vi "Set Motors.vi"(5 "Speed Multipliers":dbl=1.0, 6 "Face Joystick Axes":cluster{"X":dbl, "Y":dbl}, 7 "error in (no error)":errorcluster, 8 "Strafe Joystick Axes":cluster{"X":dbl, "Y":dbl}, 9 "Trigger Axes":cluster{"Left":dbl, "Right":dbl}, 10 "Speed Motors":T2[](array[typedef]), 11 "Position Motors":T2[](array[typedef])) -> (4 "error out":errorcluster)   [LabVIEW 2015]
uses:
  <vilib>/Rock Robotics/WPI/MotorControl/WPI_MotorControlDeviceRef.ctl
  <vilib>/Rock Robotics/WPI/MotorControl/WPI_MotorControlType.ctl
  <vilib>/Rock Robotics/SystemInterfaces/DIO/FPGA_DIOPWMChannel.ctl
  <vilib>/Rock Robotics/WPI/PWM/WPI_PWMDeadband.ctl
  <vilib>/Rock Robotics/WPI/CAN/Jaguar/SubVIs/WPI_CANJaguar_ControlMode.ctl
  <vilib>/Rock Robotics/WPI/CAN/TalonSRX/WPI_CANTalonSRX_APIControlMode.ctl
  Swerve Drive Published Globals.vi
  <vilib>/addons/control/pid/pid.llb/PID Control Input Filter (DBL).vi
  <vilib>/addons/control/pid/pid.llb/PID (DBL).vi
  <vilib>/addons/control/pid/NI_PID_pid.lvlib
panel:
  in  "Max Wheel Speed":dbl=20000.0
  in  "Angle (radians; 0 = right)":dbl
  in  "Face PID Gains":T1 {"derivative time (Td, min)" format="%.3f"; "integral time (Ti, min)" format="%.3f"; "proportional gain (Kc)" format="%.3f"}
  out "Speed Chart":cluster{dbl, "Encoder Velocity":dbl}[](graph)
  out "Position Chart":cluster{dbl, "Encoder Velocity":dbl}[](graph)
  out "Speed Cluster":T9 {"RR Speed" scale=-1.0..1.0; "RL Speed" scale=-1.0..1.0; "FR Speed" scale=-1.0..1.0; "FL Speed" scale=-1.0..1.0}
  out "Angle Cluster":T10 {"FL Angle" scale=3.1416..-3.1416; "FR Angle" scale=3.1416..-3.1416; "RR Angle" scale=3.1416..-3.1416; "RL Angle" scale=3.1416..-3.1416}
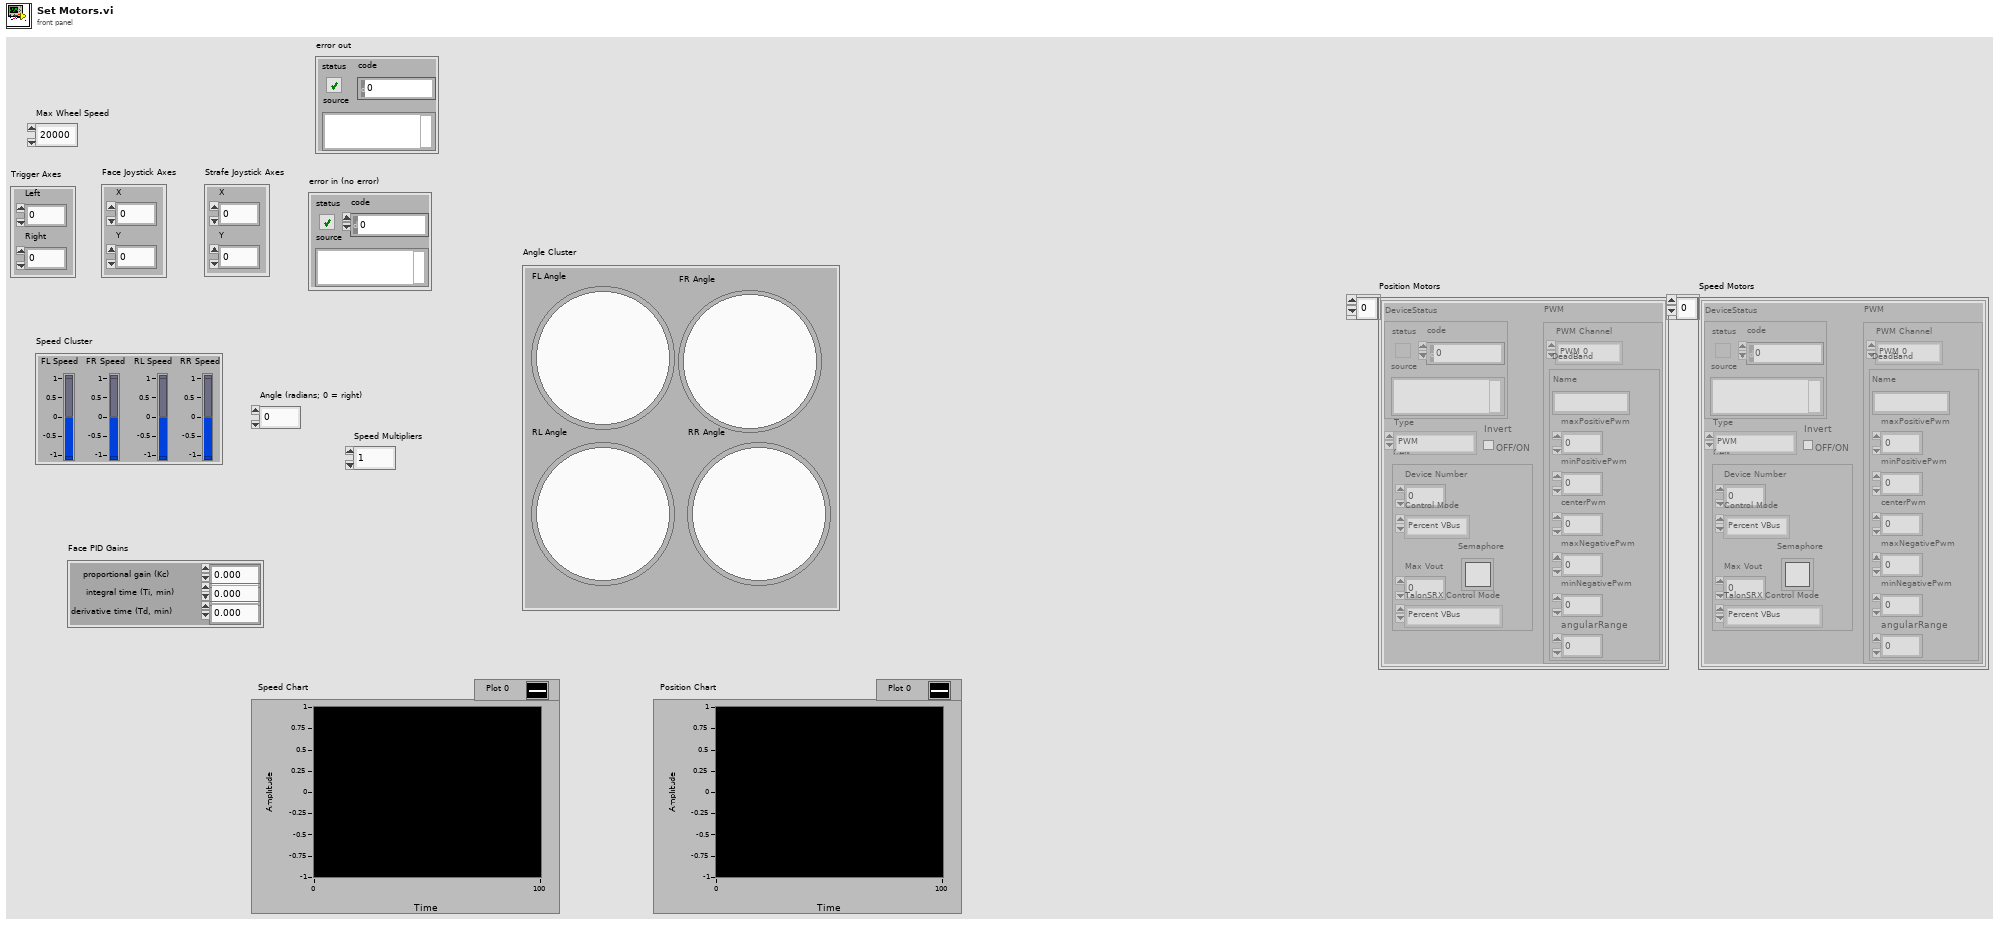
[diagram p1: front panel]
types:
  T1 = cluster{"proportional gain (Kc)":dbl, "integral time (Ti, min)":dbl, "derivative time (Td, min)":dbl}
  T2 = typedef "WPI_MotorControlDeviceRef.ctl" = cluster{"DeviceStatus":errorcluster, "Type":T3, "PWM":cluster{"PWM Channel":T4, "DeadBand":T5}, "CAN":cluster{"Device Number":u8, "Control Mode":T6, "Semaphore":T7, "Max Vout":dbl, "TalonSRX Control Mode":T8}, "Invert":bool}
  T3 = typedef "WPI_MotorControlType.ctl" = enum16{"PWM", "CAN", "CANTalonSRX"}
  T4 = typedef "FPGA_DIOPWMChannel.ctl" = enum8{"PWM 0", "PWM 1", "PWM 2", "PWM 3", "PWM 4", "PWM 5", "PWM 6", "PWM 7", "PWM 8", "PWM 9", "PWM MXP 0", "PWM MXP 1", "PWM MXP 2", "PWM MXP 3", "PWM MXP 4", "PWM MXP 5", "PWM MXP 6", "PWM MXP 7", "PWM MXP 8", "PWM MXP 9", "Invalid"}
  T5 = typedef "WPI_PWMDeadband.ctl" = cluster{"Name":string, "maxPositivePwm":i32, "minPositivePwm":i32, "centerPwm":i32, "maxNegativePwm":i32, "minNegativePwm":i32, "angularRange":u16}
  T6 = typedef "WPI_CANJaguar_ControlMode.ctl" = enum8{"Percent VBus", "Current", "Speed", "Position", "Voltage"}
  T7 = typedef "Semaphore RefNum" = refnum<k1>
  T8 = typedef "WPI_CANTalonSRX_APIControlMode.ctl" = enum8{"Percent VBus", "Speed", "Position", "Slave", "Unchanged / Invalid", "Voltage Compensation", "Current"}
  T9 = cluster{"FL Speed":dbl, "FR Speed":dbl, "RL Speed":dbl, "RR Speed":dbl}
  T10 = cluster{"FL Angle":dbl, "FR Angle":dbl, "RL Angle":dbl, "RR Angle":dbl}
  T11 = cluster{"[0]":dbl, "[1]":dbl, "[2]":dbl, "[3]":dbl}
  T12 = typedef "WPI_CANTalonSRX_GlobalStatus.ctl" = cluster{"Applied Throttle":dbl, "Module Enabled":bool, "CAN Error":errorcluster, "Closed Loop Error":dbl, "Forward Limit Switch Closed":bool, "Reverse Limit Switch Closed":bool, "Sensor Position":dbl, "Sensor Velocity":dbl, "Current":dbl, "Sticky Fault - Over Temp":bool, "Sticky Fault - Under Voltage":bool, "Sticky Fault - Forward Limit":bool, "Sticky Fault - Reverse Limit":bool, "Sticky Fault - Forward Soft Limit":bool, "Sticky Fault - Reverse Soft Limit":bool, "Brake is Enabled":bool, "Encoder Position":dbl, "Encoder Velocity":dbl, "Encoder Index Count":dbl, "Encoder A Pin State":bool, "Encoder B Pin State":bool, "Encoder Index Pin State":bool, "Analog In":dbl, "Analog In Velocity":dbl, "Temperature (C)":dbl, "Battery Voltage":dbl}
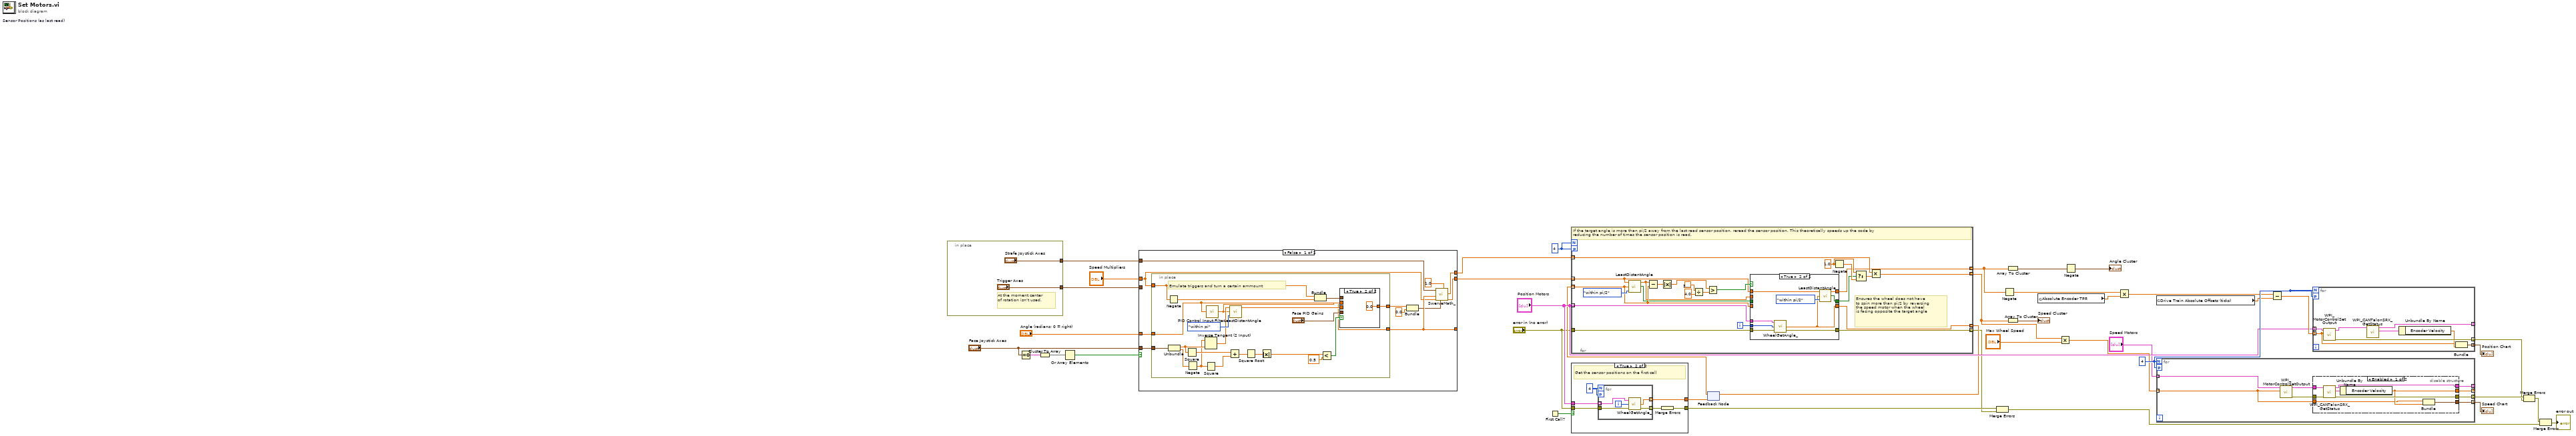
[diagram p0: block diagram]
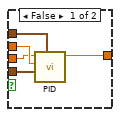
[diagram p4: hidden frame]
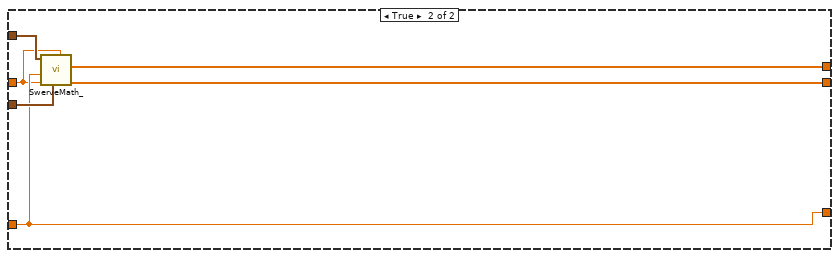
[diagram p5: hidden frame]
diagram:
  w27 = 4
  w39 = 4
  n1 = in-place {
    in-place-border: ["Strafe Joystick Axes"] -> w9
    in-place-border: ["Trigger Axes"] -> w5
    # "At the moment center\nof rotation isn't used."
  }
  n2 = Equal To 0?(x="Face Joystick Axes") -> (x = 0?=w30:cluster{"X":bool, "Y":bool})
  n3 = Cluster To Array(cluster=w30) -> (array=w28:bool[])
  n4 = Or Array Elements(Boolean array=w28) -> (logical OR=w29:bool)
  n5 = case shown="False" w29 {
    tunnel: "Face Joystick Axes" -> [w53 _]
    tunnel: [w48 w84] -> _
    tunnel: "Angle (radians; 0 = right)" -> [w52 w84]
    tunnel: w9 -> [w49 w85]
    tunnel: [w46 w83] -> w7
    tunnel: [w45 w82] -> w8
    tunnel: "Speed Multipliers" -> [w43 w81]
    tunnel: w5 -> [_ w86]
    frame False {
      n6 = in-place {
        in-place-border: [w74] -> w51
        in-place-border: [w55] -> w48
        in-place-border: w53 -> [w57]
        in-place-border: w52 -> [w55]
        in-place-border: w43 -> [w54]
        # "Emulate triggers and turn a certain ammount"
        n7 = Negate(x=w54) -> (-x=w63:dbl)
        n8 = Unbundle(w57) -> ("X"=w68:dbl, "Y"=w67:dbl)
        n9 = Square(x=w68) -> (x^2=w72:dbl)
        n10 = Negate(x=w67) -> (-x=w64:dbl)
        n11 = Inverse Tangent (2 Input)(1:w68, 2:w64) -> (0:w60:dbl)
        n12 = Square(x=w64) -> (x^2=w71:dbl)
        n13 = call-poly <vilib>:"PID Control Input Filter.vi"("input"=w55) -> ("output"=w58:dbl)  [unwired: 4 in]
        n14 = Add(x=w72, y=w71) -> (x+y=w70:dbl)
        n15 = call "LeastDistantAngle.vi"("Enum"=enum16{"within pi", "within pi/2"}."within pi", "Current angle"=w58, "target angle (between pi and -pi)"=w60) -> ("output angle"=w56:dbl)  [unwired: 2 out]
        n16 = Square Root(x=w70) -> (sqrt(x)=w69:dbl)
        n17 = Absolute Value(x=w69) -> (abs(x)=w65:dbl)
        n18 = Bundle("Speed Multipliers"=w54, w63) -> (w62:cluster{"Speed Multipliers":dbl, dbl})  [unwired: 1 in]
        n19 = Less?(x=w65, y=0.5) -> (x < y?=w59:bool)
        n20 = case shown="True" w59 {
          tunnel: [w79 0.0 ("output")] -> w74
          tunnel: "Face PID Gains" -> [w78 _]
          tunnel: w62 -> [w77 _]
          tunnel: w58 -> [w76 _]
          tunnel: w56 -> [w75 _]
          frame False {
            n21 = call-poly <vilib>:"PID.vi"("output range"=w77, "PID gains"=w78, "process variable"=w76, "setpoint"=w75) -> ("output"=w79:dbl)  [unwired: 6 in, 1 out]
          }
          frame True {
          }
        }
      }
      n22 = Bundle("output"=w51, 0.0) -> (w47:cluster{"output":dbl, dbl})  [unwired: 1 in]
      n23 = call "SwerveMath_.vi"("Rotation Multiplier"=1.0, "Trigger Axes/Turn Speed"=w47, "Strafe Multiplier"=w43, "Angle (radians; 0 = right)"=w48, "Strafe Joystick Axes"=w49) -> ("Motor Angles"=w45:dbl[], "Motor Speeds"=w46:dbl[])  [unwired: 4 in]
    }
    frame True {
      n24 = call "SwerveMath_.vi"("Rotation Multiplier"=w81, "Trigger Axes/Turn Speed"=w86, "Strafe Multiplier"=w81, "Angle (radians; 0 = right)"=w84, "Strafe Joystick Axes"=w85) -> ("Motor Angles"=w82:dbl[], "Motor Speeds"=w83:dbl[])  [unwired: 4 in]
    }
  }
  n25 = First Call?() -> (First Call?: T/F=w24:bool)
  n26 = case shown="True" w24 {
    tunnel: "error in (no error)" -> [w87 w93]
    tunnel: [w87 w92] -> w23
    tunnel: "Position Motors" -> [_ w91]
    tunnel: [_ w90] -> w20
    frame False {
    }
    frame True {
      w88 = 4
      # "Get the sensor positions on the first call"
      n27 = for {
        N: w88 -> [_]
        tunnel: [w97] -> w90 mode=indexing
        tunnel: w93 -> [w98]
        tunnel: [w96] -> w89 mode=indexing
        workers-P: w88 -> [_]
        tunnel: w91 -> [w95] mode=indexing
        i -> [w94]
        n28 = call "WheelGetAngle_.vi"("error in (no error)"=w98, "Wheel"=w94, "CAN Talon SRX Ref"=w95) -> ("error out"=w96:errorcluster, "Sensor Position (rad)"=w97:dbl)  [unwired: 1 out]
      }
      n29 = Merge Errors(w89) -> (w92:errorcluster)
    }
  }
  n30 = feedback #1 "Sensor Positions (as last read)"(w20) -> (w25:dbl[])
  n31 = for {
    N: w27 -> [_]
    workers-P: w27 -> [_]
    tunnel: [w121] -> w26 mode=indexing
    tunnel: w8 -> [w99] mode=indexing
    tunnel: w25 -> [w110] mode=indexing
    tunnel: "error in (no error)" -> [w120]
    tunnel: [w119] -> w21 mode=indexing
    tunnel: "Position Motors" -> [w117] mode=indexing
    tunnel: w7 -> [w105] mode=indexing
    tunnel: [w104] -> w18 mode=indexing
    tunnel: [w102] -> w12 mode=indexing
    i -> [w116]
    w108 = 1.0 ("t")
    # "Ensures the wheel does not have\nto spin more than pi/2 by reversing\nthe speed motor when the wheel\nis facing opposite the target angle"
    # "If the target angle is more than pi/2 away from the last read sensor position, reread the sensor position. This theoretically speeds up the code by\nreducing the number of times the sensor position is read."
    n32 = call "LeastDistantAngle.vi"("Enum"=enum16{"within pi", "within pi/2"}."within pi/2", "Current angle"=w110, "target angle (between pi and -pi)"=w99) -> ("Reverse?"=w100:bool, "output angle"=w103:dbl)  [unwired: 1 out]
    n33 = Subtract(x=w103, y=w110) -> (x-y=w109:dbl)
    n34 = Absolute Value(x=w109) -> (abs(x)=w115:dbl)
    n35 = Divide(x=3.141592653589793, y=4.0) -> (x/y=w112:dbl)
    n36 = Greater?(x=w115, y=w112) -> (0:w118:bool)
    n37 = case shown="True" w118 {
      tunnel: [w125 w126] -> w121
      tunnel: w110 -> [w125 _]
      tunnel: w120 -> [w124 w128]
      tunnel: [w124 w127] -> w119
      tunnel: w117 -> [_ w130]
      tunnel: w116 -> [_ w129]
      tunnel: w103 -> [w123 _]
      tunnel: [w123 w131] -> w102
      tunnel: [w122 w132] -> w101
      tunnel: w100 -> [w122 _]
      tunnel: w99 -> [_ w133]
      frame False {
      }
      frame True {
        n38 = call "WheelGetAngle_.vi"("error in (no error)"=w128, "Wheel"=w129, "CAN Talon SRX Ref"=w130) -> ("error out"=w127:errorcluster, "Sensor Position (rad)"=w126:dbl)  [unwired: 1 out]
        n39 = call "LeastDistantAngle.vi"("Enum"=enum16{"within pi", "within pi/2"}."within pi/2", "Current angle"=w126, "target angle (between pi and -pi)"=w133) -> ("Reverse?"=w132:bool, "output angle"=w131:dbl)  [unwired: 1 out]
      }
    }
    n40 = Negate(x=w108) -> (-x=w107:dbl)
    n41 = Select(t=w108, s=w101, f=w107) -> (s? t:f=w106:dbl)
    n42 = Multiply(x=w105, y=w106) -> (x*y=w104:dbl)
  }
  n43 = feedback-in #1(w26) -> ()
  n44 = Merge Errors(w23, w21) -> (w3:errorcluster)
  n45 = Negate(x=w12) -> (-x=w11:dbl[])
  n46 = Array To Cluster(array=w12) -> (cluster=w13:T11)
  n47 = Array To Cluster(array=w18) -> (cluster=→"Speed Cluster":T11)
  n48 = global read "Swerve Drive Published Globals.vi" "Absolute Encoder TPR"() -> (w17:dbl)
  n49 = Multiply(x=w18, y="Max Wheel Speed") -> (x*y=w34:dbl[])
  n50 = Negate(x=w13) -> (-x=→"Angle Cluster":T11)
  n51 = Multiply(x=w11, y=w17) -> (x*y=w15:dbl[])
  n52 = global read "Swerve Drive Published Globals.vi" "Drive Train Absolute Offsets (ticks)"() -> (w16:dbl[])
  n53 = for {
    N: w39 -> [_]
    tunnel: [w140] -> w40 mode=indexing
    workers-P: w39 -> [_]
    tunnel: "Speed Motors" -> [w142] mode=indexing
    tunnel: [w138] -> _ mode=indexing
    tunnel: [w137] -> w37 mode=indexing
    tunnel: w34 -> [w136] mode=indexing
    tunnel: [w135] -> _ mode=indexing
    n54 = call <vilib>:"WPI_MotorControlSetOutput.vi"("Output"=w136, "MotorControlDevRef"=w142) -> ("error out"=w141:errorcluster, "MotorControlDevRef"=w139:T2)  [unwired: 7 in, 1 out]
    n55 = disable-structure shown="Enabled" {
      disable-tunnel: w141 -> [w150 w151]
      disable-tunnel: [w149 w151] -> w140
      disable-tunnel: w139 -> [w148 _]
      disable-tunnel: [w146 _] -> w138
      disable-tunnel: [w144 _] -> w137
      disable-tunnel: w136 -> [w145 _]
      disable-tunnel: [w143 _] -> w135
      frame Enabled {
        n56 = call <vilib>:"WPI_CANTalonSRX_GetStatus.vi"("error in (no error)"=w150, "CAN Talon SRX Ref"=w148) -> ("error out"=w149:errorcluster, "Talon SRX Status"=w147:T12, "CAN Talon SRX Ref Out"=w143:T2)  [unwired: 7 in]
        n57 = Unbundle By Name(w147) -> ("Encoder Velocity"=w146:dbl)
        n58 = Bundle(w145, "Encoder Velocity"=w146) -> (w144:cluster{dbl, "Encoder Velocity":dbl})  [unwired: 1 in]
      }
      frame Disabled {
      }
    }
  }
  "Speed Chart" <- w37
  n59 = Subtract(x=w15, y=w16) -> (x-y=w35:dbl[])
  n60 = for {
    N: w39 -> [_]
    workers-P: w39 -> [_]
    tunnel: "Position Motors" -> [w159] mode=indexing
    tunnel: w35 -> [w154] mode=indexing
    tunnel: [w158] -> w38 mode=indexing
    tunnel: [w153] -> w36 mode=indexing
    tunnel: [w152] -> _ mode=indexing
    n61 = call <vilib>:"WPI_MotorControlSetOutput.vi"("Output"=w154, "MotorControlDevRef"=w159) -> ("error out"=w158:errorcluster, "MotorControlDevRef"=w156:T2)  [unwired: 7 in, 1 out]
    n62 = call <vilib>:"WPI_CANTalonSRX_GetStatus.vi"("CAN Talon SRX Ref"=w156) -> ("Talon SRX Status"=w157:T12, "CAN Talon SRX Ref Out"=w152:T2)  [unwired: 8 in, 1 out]
    n63 = Unbundle By Name(w157) -> ("Encoder Velocity"=w155:dbl)
    n64 = Bundle(w154, "Encoder Velocity"=w155) -> (w153:cluster{dbl, "Encoder Velocity":dbl})  [unwired: 1 in]
  }
  "Position Chart" <- w36
  n65 = Merge Errors(w40, w38) -> (w2:errorcluster)
  n66 = Merge Errors(w2, w3) -> (→"error out":errorcluster)
